vi "Close Connections.vi"(10 "netw Variable References":T1) -> ()   [LabVIEW 2014]
uses:
  Controls/pR Variable References.ctl
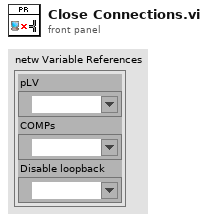
[diagram p1: front panel]
types:
  T1 = typedef "pR Variable References.ctl" = cluster{"pLV":refnum<k21>, "COMPs":refnum<k21>, "Disable loopback":refnum<k21>}
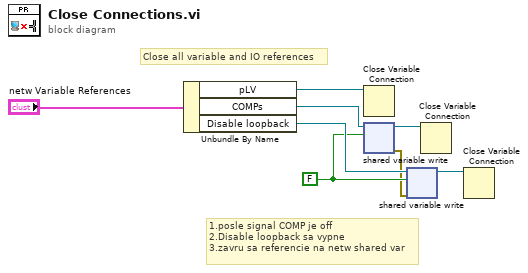
[diagram p0: block diagram]
diagram:
  w3 = FALSE ("data in")
  # "1.posle signal COMP je off\n2.Disable loopback sa vypne \n3.zavru sa referencie na netw shared var"
  # "Close all variable and IO references"
  n1 = Unbundle By Name("netw Variable References") -> ("pLV"=w8:refnum<k21>, "COMPs"=w6:refnum<k21>, "Disable loopback"=w4:refnum<k21>)
  n2 = Close Variable Connection(11:w8) -> ()  [unwired: 1 in, 1 out]
  n3 = shared-variable-write(w6, w3) -> (w5:refnum<k21>, w1:errorcluster)  [unwired: 1 in]
  n4 = shared-variable-write(w4, w1, w3) -> (w2:refnum<k21>)  [unwired: 1 out]
  n5 = Close Variable Connection(11:w5) -> ()  [unwired: 1 in, 1 out]
  n6 = Close Variable Connection(11:w2) -> ()  [unwired: 1 in, 1 out]
